vi "reciver.vi"() -> ()   [LabVIEW 2021]
panel:
  out "BeagleBonePort":i32=8089
  out "BeagleBoneIP":string="192.168.0.21"
  out "Dados Recebidos":dbl format="%+09.3f"
  out "Waveform Graph":dbl[](graph)
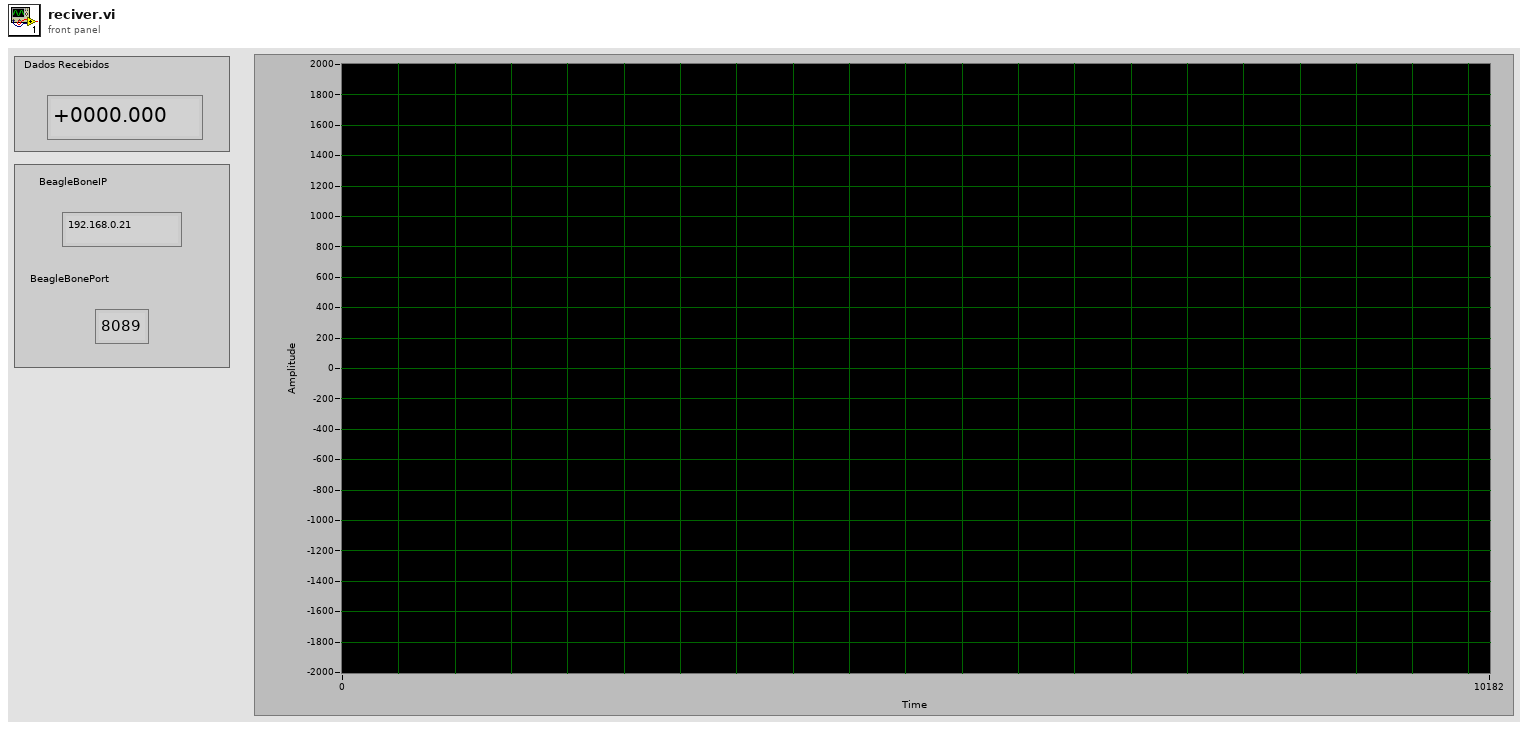
[diagram p1: front panel]
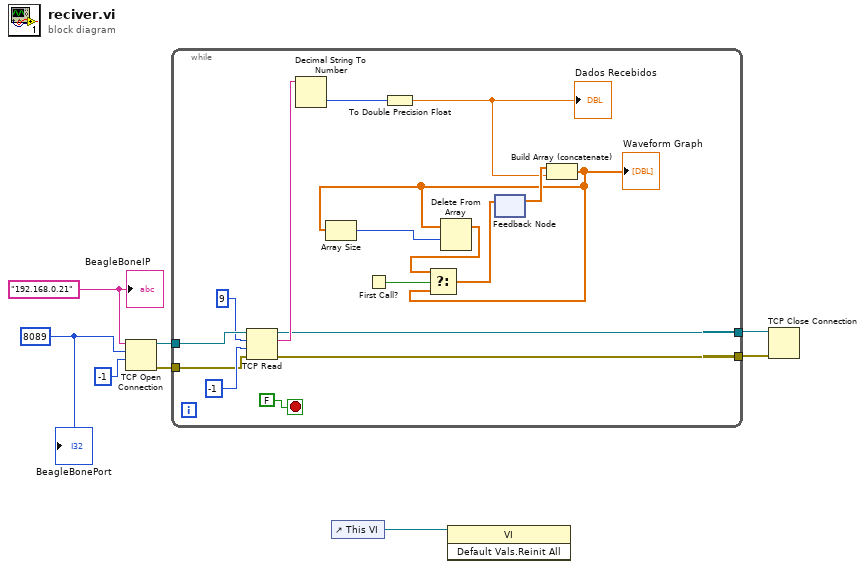
[diagram p0: block diagram]
diagram:
  w4 = "192.168.0.21"
  w8 = 8089
  n1 = TCP Open Connection(address=w4, remote port or service name=w8, timeout ms (60000)=-1) -> (connection ID=w6:refnum<k5>, error out=w5:errorcluster)  [unwired: 2 in]
  n2 = while {
    tunnel: w6 -> [w23]
    tunnel: w5 -> [w22]
    tunnel: [w19] -> w3
    tunnel: [w18] -> w2
    stop <- FALSE stop-if-true
    n3 = TCP Read(connection ID=w23, bytes to read=9, error in (no error)=w22, 9:-1) -> (connection ID out=w19:refnum<k5>, data out=w20:string, error out=w18:errorcluster)  [unwired: 1 in]
    n4 = Decimal String To Number(string=w20) -> (number=w11:i32)  [unwired: 2 in, 1 out]
    n5 = First Call?() -> (First Call?: T/F=w12:bool)
    n6 = To Double Precision Float(number=w11) -> (double precision float=w10:dbl)
    "Dados Recebidos" <- w10
    n7 = feedback #1() -> (w13:dbl[])  [unwired: 1 in]
    n8 = Build Array (concatenate)(w13, w10) -> (w9:dbl[])
    "Waveform Graph" <- w9
    n9 = Array Size(array=w9) -> (size(s)=w15:i32)
    n10 = Delete From Array(array=w9, length=w15) -> (array with subset deleted=w14:dbl[])  [unwired: 1 in, 1 out]
    n11 = Select(t=w14, s=w12, f=w9) -> (s? t:f=w16:dbl[])
    n12 = feedback-in #1(w16) -> ()
  }
  n13 = control-ref of="This VI"() -> (w1:refnum<vi>)
  n14 = invoke class="VI" method="Default Vals.Reinit All"(reference=w1) -> ()  [unwired: 2 in, 3 out]
  n15 = TCP Close Connection(connection ID=w3, error in (no error)=w2) -> ()  [unwired: 1 in, 2 out]
  "BeagleBoneIP" <- w4
  "BeagleBonePort" <- w8
